vi "Print.vi"() -> ()   [LabVIEW 2011]
uses:
  <vilib>/Utility/NIReport.llb/NI_ReportGenerationCore.lvlib
panel:
  out "default printer":string caption="默认打印机"
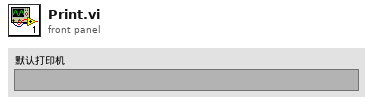
[diagram p1: front panel]
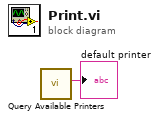
[diagram p0: block diagram]
diagram:
  n1 = call <vilib>:"Query Available Printers.vi"() -> ("default printer"=→"default printer":string)  [unwired: 9 in, 2 out]
